vi "Solve CxBand Linear Equations (Single right hand).vi"(8 "Known Vector":cdb[](array[numeric]) format="%.2f", 9 "# of super-diagonal":i32, 10 "# of sub-diagonal":i32, 11 "Banded Matrix":cdb[][](array[numeric]) format="%.2f") -> (0 "error":i32, 3 "Solution Vector":cdb[](array[numeric]) format="%.2f")   [LabVIEW 2020, in "NI_AALPro.lvlib"]
doc: "Computes the solution to the system of linear equations AX=Y with a band coefficient matrix A and single or multiple right-hand sides Y."
uses:
  NI_AALPro.lvlib
  <resource>/lvanlys.dll
panel:
  # "Solve Complex Band Linear Equations"
  # "Must be in band storage"
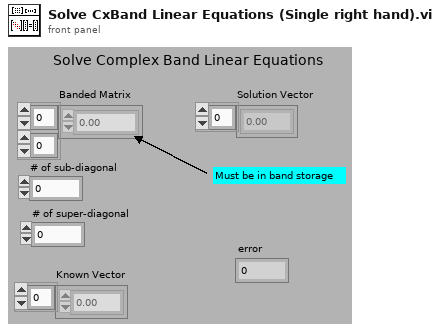
[diagram p1: front panel]
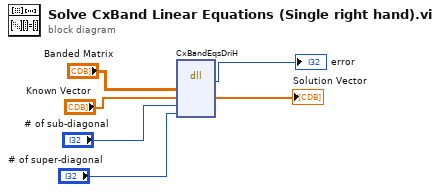
[diagram p0: block diagram]
diagram:
  n1 = dll-call lib="C:/Program Files (x86)/National Instruments/LabVIEW 2020/resource/lvanlys.*" fn="CxBandEqsDriH"("Banded Matrix"="Banded Matrix", "Known Vector"="Known Vector", "kl"="# of sub-diagonal", "ku"="# of super-diagonal") -> (→"error":i32, "Known Vector"=→"Solution Vector":cdb[])  [unwired: 6 in, 2 out]
